vi "ChassiDriveUpdate.vi"   [LabVIEW 2014, in "ChassisLib.lvlib"]
uses:
  ChassisLib.lvlib
  ChassisRefs.ctl
types:
  T1 = typedef "ChassisLib.lvlib/ChassisRefs.ctl" = enum16{"RobotDrive"}
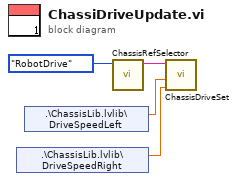
[diagram p0: block diagram]
diagram:
  n1 = shared-variable ".\\ChassisLib.lvlib\\DriveSpeedRight"() -> (w4:dbl)  [unwired: 1 in, 1 out]
  n2 = shared-variable ".\\ChassisLib.lvlib\\DriveSpeedLeft"() -> (w3:dbl)  [unwired: 1 in, 1 out]
  n3 = call "ChassisRefSelector.vi"("Enum 2"=ChassisRefs."RobotDrive") -> ("String"=w1:string)  [unwired: 10 in]
  n4 = call "ChassisDriveSet.vi"("Right axis value"=w4, "Left axis value"=w3, "DriveRef"=w1) -> ()  [unwired: 9 in]
